vi "Start Sync.vi"(8 "error in (no error)":errorcluster, 11 "OOP Server in":refnum<class "OOP Server.lvclass">) -> (0 "error out":errorcluster, 3 "OOP Server out":refnum<class "OOP Server.lvclass">)   [LabVIEW 2019, in "OOP Server.lvclass"]
uses:
  OOP Server.lvclass
  RPC Messages/QueryReponse/QueryResponse_Data.ctl
  gRPC interface/Server API/typeDefs/grpcId.ctl
  gRPC interface/gprc-lvsupport.lvlib
  RPC Messages/ServerEvent/ServerEvent_Data.ctl
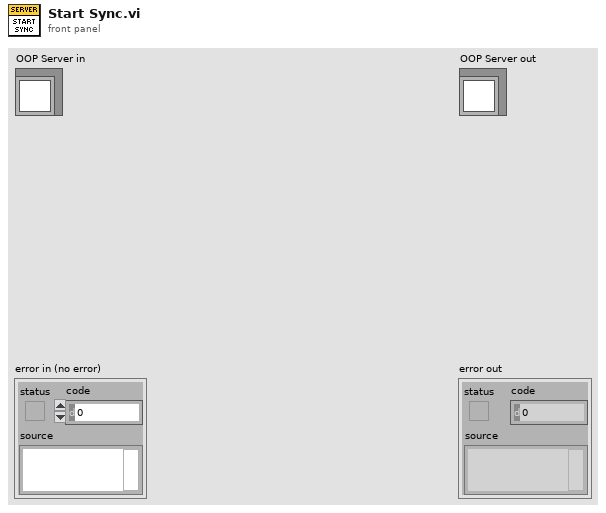
[diagram p1: front panel]
types:
  T1 = typedef "OOP Server.lvclass/ServerEvent_Data.ctl" = cluster{"eventData":string, "serverId":i32, "status":i32}
  T2 = typedef "OOP Server.lvclass/QueryResponse_Data.ctl" = cluster{"message":string, "status":i32}
  T3 = typedef "gprc-lvsupport.lvlib/grpcId.ctl" = u64
  T4 = typedef "OOP Server.lvclass/Server gRPC UEs.ctl" = cluster{"Invoke gRPC UEs":T5, "Query gRPC UEs":T5, "Register gRPC UEs":T5}
  T5 = typedef "gprc-lvsupport.lvlib/gRPCId Cluster UE.ctl" = refnum<user-event>
  T6 = typedef "OOP Server.lvclass/InvokeRequest_Data.ctl" = cluster{"command":string, "parameter":string}
  T7 = typedef "OOP Server.lvclass/QueryRequest_Data.ctl" = cluster{"query":string}
  T8 = typedef "OOP Server.lvclass/RegistrationRequest_Data.ctl" = cluster{"eventName":string}
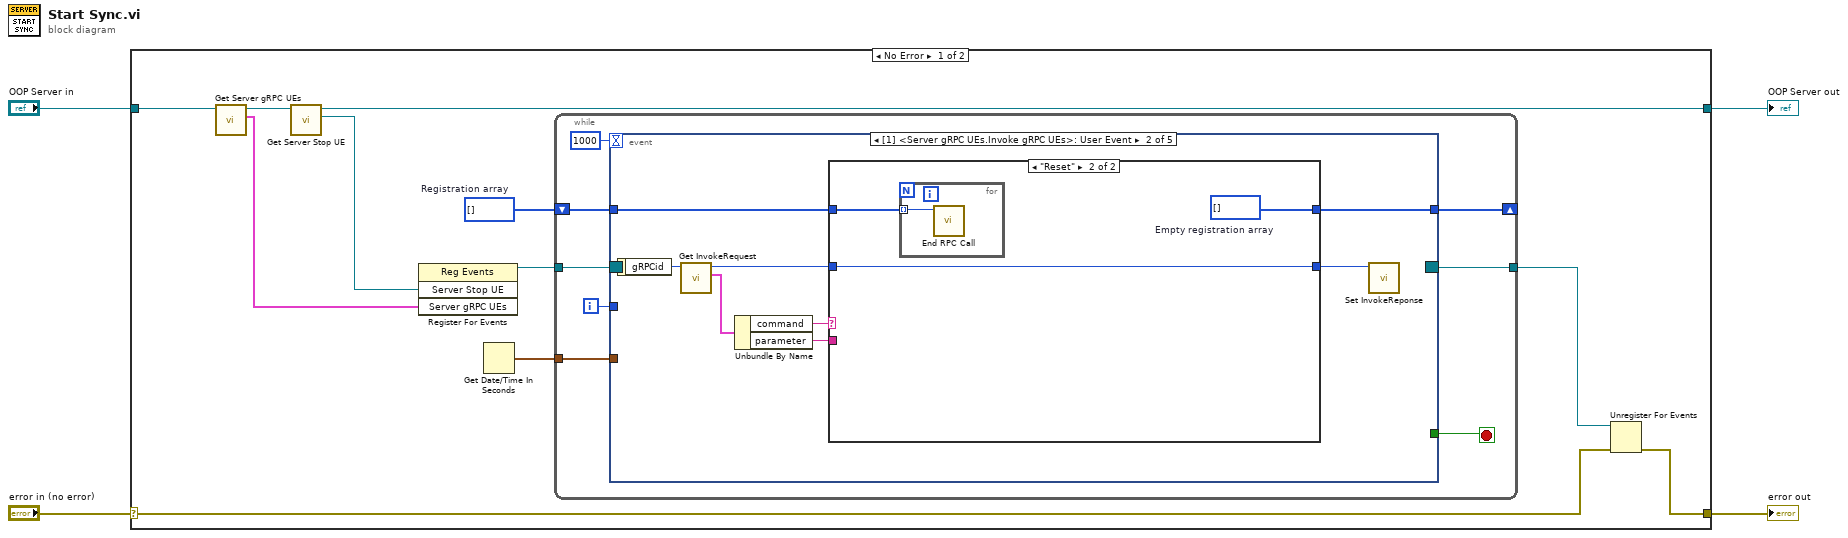
[diagram p0: block diagram]
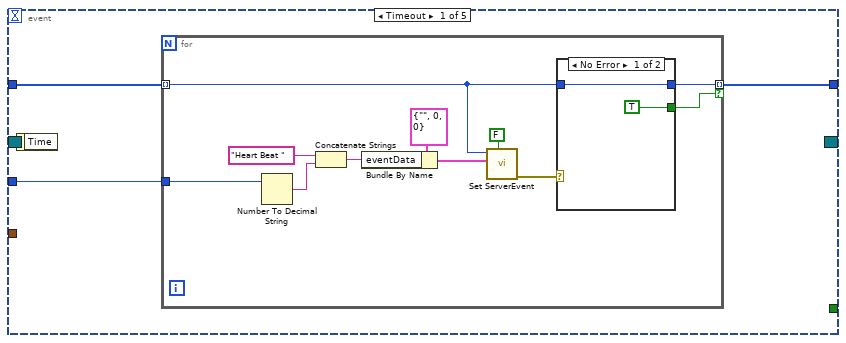
[diagram p2: hidden frame]
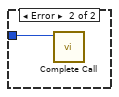
[diagram p3: hidden frame]
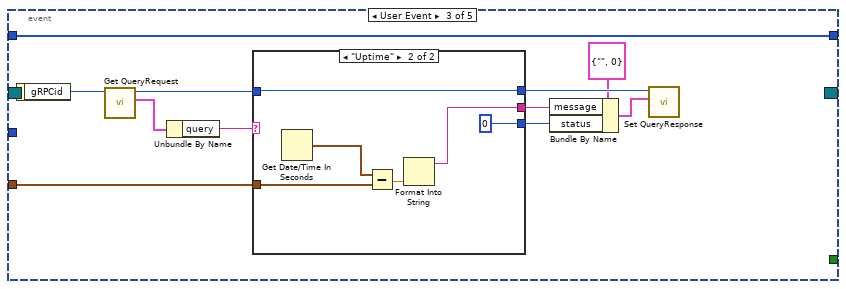
[diagram p5: hidden frame]
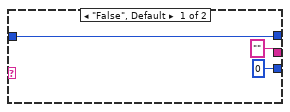
[diagram p6: hidden frame]
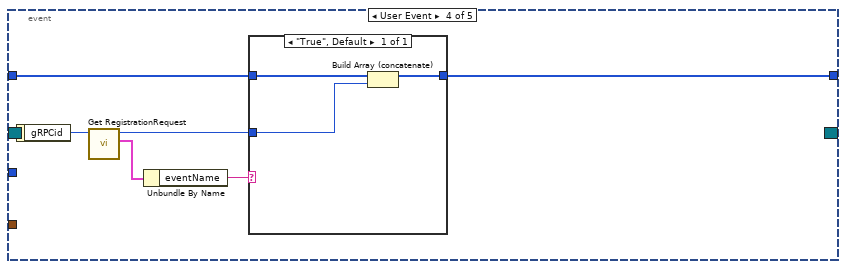
[diagram p7: hidden frame]
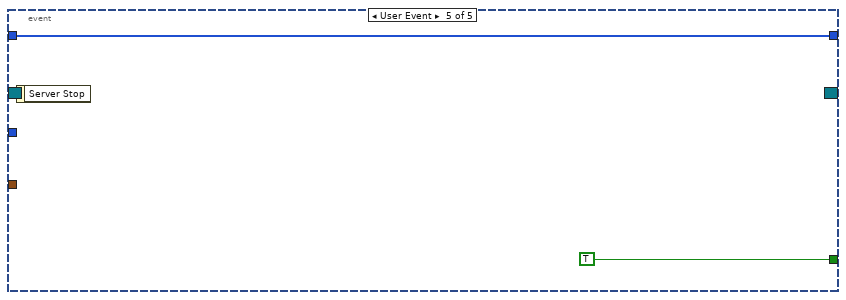
[diagram p8: hidden frame]
diagram:
  n1 = case shown="No Error" "error in (no error)" {
    selector: "error in (no error)" -> [w8 w87]
    tunnel: [w7 w87] -> w3
    tunnel: [w11 w86] -> w1
    tunnel: "OOP Server in" -> [w15 w86]
    frame No Error {
      w5 = T3[] []  # Registration array
      n2 = call "Get Server gRPC UEs.vi"("OOP Server in"=w15) -> ("Server gRPC UEs"=w12:T4, "OOP Server out"=w14:refnum<class "OOP Server.lvclass">)  [unwired: 9 in]
      n3 = call "Get Server Stop UE.vi"("OOP Server in"=w14) -> ("Server Stop UE"=w13:refnum<user-event>, "OOP Server out"=w11:refnum<class "OOP Server.lvclass">)  [unwired: 9 in]
      n4 = register-events(w13, w12) -> (reference out=w10:refnum<event-registration>)  [unwired: 2 in, 1 out]
      n5 = Get Date/Time In Seconds() -> (seconds since 1Jan1904=w6:timestamp)
      n6 = while {
        tunnel: w10 -> [w23]
        tunnel: [w21] -> w9
        tunnel: w6 -> [w20]
        shift-right: [w18] -> _
        shift-left: w5 -> [w19]
        i -> [w17]
        stop <- w22 stop-if-true
        n7 = event shown="[1] <Server gRPC UEs.Invoke gRPC UEs>: User Event" {
          selector: w23 -> [_ _ _ _ _]
          dyn-events: [_ _ _ _ _] -> w21
          timeout: 1000 -> [_ _ _ _ _]
          tunnel: [_ _ _ _ TRUE] -> w22
          tunnel: w20 -> [_ _ w61 _ _]
          tunnel: w19 -> [w26 w42 w55 w76 w84]
          tunnel: [w25 w41 w55 w75 w84] -> w18
          tunnel: w17 -> [w24 _ _ _ _]
          event Timeout {
            n8 = event-data() -> ()  [unwired: 1 in, 1 out]
            n9 = for {
              tunnel: w26 -> [w28] mode=indexing
              tunnel: [w30] -> w25 mode=indexing if=w29
              tunnel: w24 -> [w32]
              n10 = Number To Decimal String(number=w32) -> (decimal integer string=w37:string)  [unwired: 1 in]
              n11 = Concatenate Strings("Heart Beat " ("eventdata"), w37) -> (w34:string)
              n12 = Bundle By Name(cluster=T1 {"eventData"="", "serverId"=0, "status"=0} ("ServerEvent_Data"), "eventData"=w34) -> (w33:T1)
              n13 = call "Set ServerEvent.vi"("Complete Call (T)"=FALSE, "ServerEvent_Data"=w33, "gRPCid in"=w28) -> ("error out"=w31:errorcluster)  [unwired: 8 in]
              n14 = case shown="No Error" w31 {
                tunnel: w28 -> [w39 w40]
                tunnel: [w39 _] -> w30
                tunnel: [TRUE _] -> w29
                frame No Error {
                }
                frame Error {
                  n15 = call "Complete Call.vi"("gRPCid"=w40) -> ()  [unwired: 9 in, 1 out]
                }
              }
            }
          }
          event User Event {
            n16 = event-data() -> ("gRPCid"=w48:T3)  [unwired: 1 in]
            n17 = call "Get InvokeRequest.vi"("gRPCid"=w48) -> ("Request Data"=w47:T6, "gRPCid out"=w44:T3)  [unwired: 8 in, 1 out]
            n18 = Unbundle By Name(w47) -> ("command"=w46:string, "parameter"=w45:string)
            n19 = case shown="\"Reset\"" w46 {
              tunnel: w45 -> [_ _]
              tunnel: w44 -> [w50 w53]
              tunnel: [w50 w53] -> w43
              tunnel: w42 -> [w49 w52]
              tunnel: [w49 w51] -> w41
              frame "None", Default {
              }
              frame "Reset" {
                w51 = T3[] []  # Empty registration array
                n20 = for {
                  tunnel: w52 -> [w54] mode=indexing
                  n21 = call "End RPC Call.vi"("gRPCid"=w54) -> ()  [unwired: 10 in, 1 out]
                }
              }
            }
            n22 = call "Set InvokeReponse.vi"("gRPCid"=w43) -> ()  [unwired: 10 in, 1 out]
          }
          event User Event {
            n23 = event-data() -> ("gRPCid"=w65:T3)  [unwired: 1 in]
            n24 = call "Get QueryRequest.vi"("gRPCid"=w65) -> ("Request Data"=w64:T7, "gRPCid out"=w62:T3)  [unwired: 8 in, 1 out]
            n25 = Unbundle By Name(w64) -> ("query"=w63:string)
            n26 = case shown="\"Uptime\"" w63 {
              tunnel: w62 -> [w68 w71]
              tunnel: w61 -> [_ w72]
              tunnel: [w68 w71] -> w60
              tunnel: ["" w70] -> w57
              tunnel: [0 ("status") 0 ("status")] -> w56
              frame "False", Default {
              }
              frame "Uptime" {
                n27 = Get Date/Time In Seconds() -> (seconds since 1Jan1904=w74:timestamp)
                n28 = Subtract(x=w74, y=w72) -> (x-y=w73:dbl)
                n29 = Format Into String(w73) -> (resulting string=w70:string)  [unwired: 3 in, 1 out]
              }
            }
            n30 = Bundle By Name(cluster=T2 {"message"="", "status"=0} ("QueryResponse_Data"), "message"=w57, "status"=w56) -> (w58:T2)
            n31 = call "Set QueryResponse.vi"("QueryResponse_Data"=w58, "gRPCid"=w60) -> ()  [unwired: 9 in, 1 out]
          }
          event User Event {
            n32 = event-data() -> ("gRPCid"=w80:T3)  [unwired: 1 in]
            n33 = call "Get RegistrationRequest.vi"("gRPCid in"=w80) -> ("Request Data"=w79:T8, "gRPCid out"=w77:T3)  [unwired: 8 in, 1 out]
            n34 = Unbundle By Name(w79) -> ("eventName"=w78:string)
            n35 = case shown="\"True\", Default" w78 {
              tunnel: w77 -> [w83]
              tunnel: w76 -> [w82]
              tunnel: [w81] -> w75
              frame "True", Default {
                n36 = Build Array (concatenate)(w82, w83) -> (w81:T3[])
              }
            }
          }
          event User Event {
            n37 = event-data() -> ()  [unwired: 1 in, 1 out]
          }
        }
      }
      n38 = Unregister For Events(event registration refnum=w9, error in=w8) -> (error out=w7:errorcluster)
    }
    frame Error {
    }
  }
  "error out" <- w3
  "OOP Server out" <- w1
